vi "SetSystemDefinitionPropertyValue_String.vi"(8 "error in (no error)":errorcluster, 9 "value":string, 10 "property name":string, 11 "BaseNodeType in":refnum<k24>) -> (0 "error out":errorcluster, 3 "BaseNodeType out":refnum<k24>)   [LabVIEW 2015, in "VeriStandTestUtilities.lvlib"]
uses:
  VeriStandTestUtilities.lvlib
  NationalInstruments.VeriStand.SystemStorage
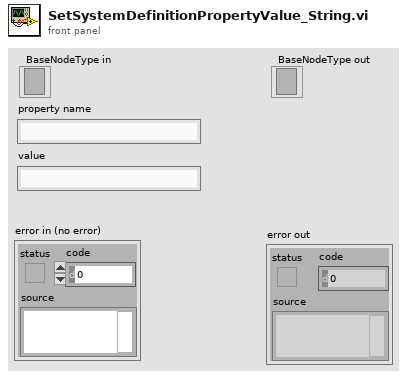
[diagram p1: front panel]
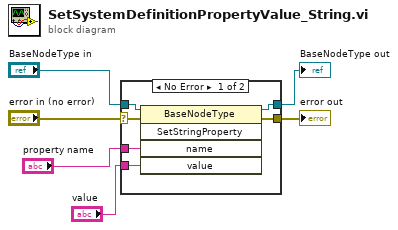
[diagram p0: block diagram]
diagram:
  n1 = case shown="No Error" "error in (no error)" {
    selector: "error in (no error)" -> [w11 w14]
    tunnel: "BaseNodeType in" -> [w12 w13]
    tunnel: "property name" -> [w10 _]
    tunnel: [w9 w13] -> w1
    tunnel: [w8 w14] -> w2
    tunnel: "value" -> [w7 _]
    frame No Error {
      n2 = invoke class="BaseNodeType" method="SetStringProperty"(reference=w12, error in=w11, "name"=w10, "value"=w7) -> (reference out=w9:refnum<k24>, error out=w8:errorcluster)  [unwired: 1 in, 3 out]
    }
    frame Error {
    }
  }
  "error out" <- w2
  "BaseNodeType out" <- w1
